vi "ReadPattern.vi"(0 "file path (dialog if empty)":path=path "/Users/zschillaci/BNL/Working/BNL_ThermomechanicalStave/SchillaciGlue/Utilities/pattern.txt") -> (1 "Relative Positions [mm]":dbl[][](array[numeric]), 2 "Line Lengths [mm]":dbl[][](array[numeric]), 3 "Line Speeds [mm/s]":dbl[][](array[numeric]), 4 "N Lines":i32[](array[numeric]))   [LabVIEW 2016]
uses:
  <vilib>/Utility/file.llb/Read Delimited Spreadsheet (DBL).vi
panel:
  out "all rows":dbl[][](array[numeric])
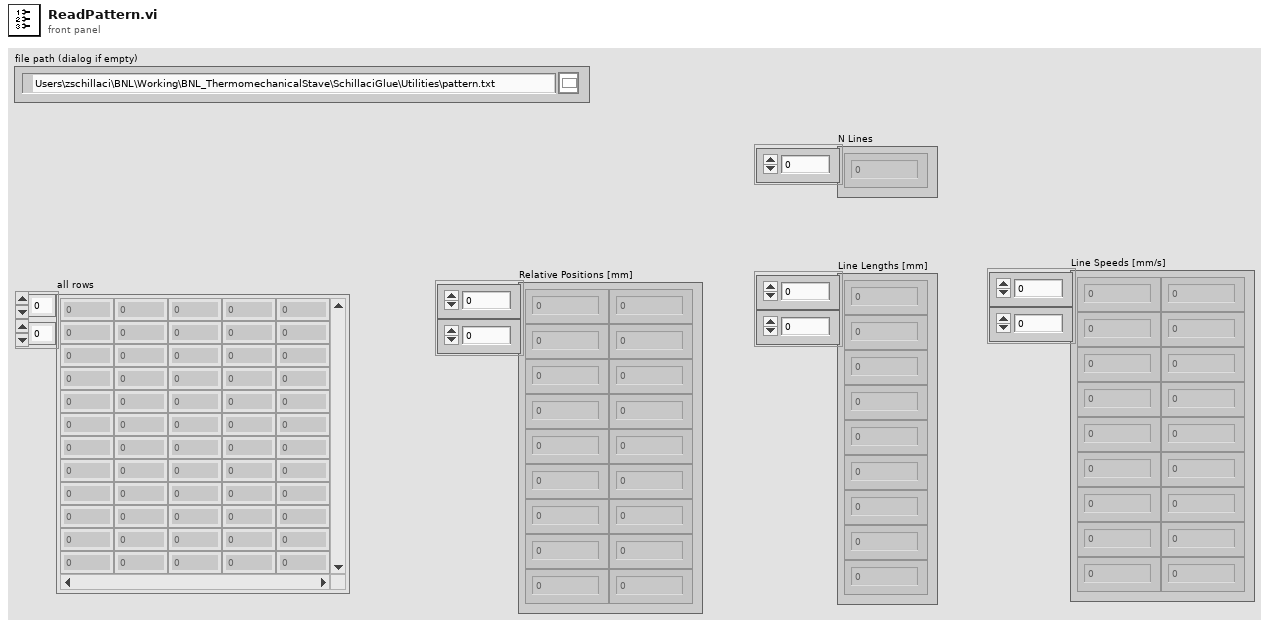
[diagram p1: front panel]
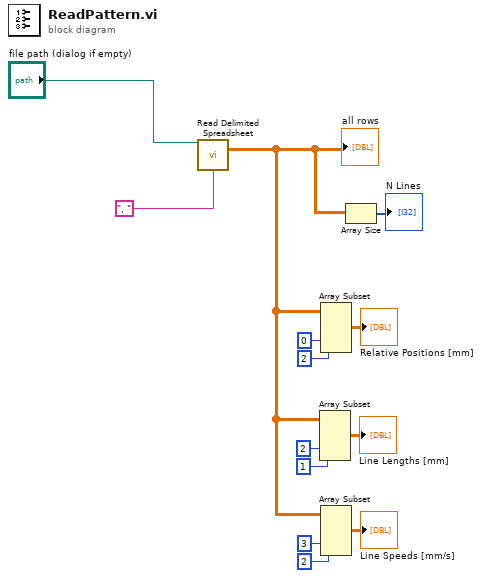
[diagram p0: block diagram]
diagram:
  n1 = call-poly <vilib>:"Read Delimited Spreadsheet.vi"("file path (dialog if empty)"="file path (dialog if empty)", "delimiter (\\t)"=", " ("delimiter (\\t)")) -> ("all rows"=w2:dbl[][])  [unwired: 8 in, 5 out]
  "all rows" <- w2
  n2 = Array Subset(array=w2, index (col)=2 ("index"), length (col)=1 ("length")) -> (→"Line Lengths [mm]":dbl[][])  [unwired: 2 in]
  n3 = Array Subset(array=w2, index (col)=0 ("index"), length (col)=2 ("length")) -> (→"Relative Positions [mm]":dbl[][])  [unwired: 2 in]
  n4 = Array Subset(array=w2, index (col)=3 ("index"), length (col)=2 ("length")) -> (→"Line Speeds [mm/s]":dbl[][])  [unwired: 2 in]
  n5 = Array Size(array=w2) -> (size(s)=→"N Lines":i32[])
